vi "SacarNivelRefTablaRef.vi"(8 "error in (no error)":errorcluster, 11 "Prueba21 in":refnum<class "Prueba21.lvclass">) -> (0 "error out":errorcluster, 3 "Prueba21 out":refnum<class "Prueba21.lvclass">)   [LabVIEW 2019, in "Prueba21.lvclass"]
uses:
  Prueba21.lvclass
  Prueba21.lvclass/Prueba21.ctl
  Prueba/Prueba.lvclass
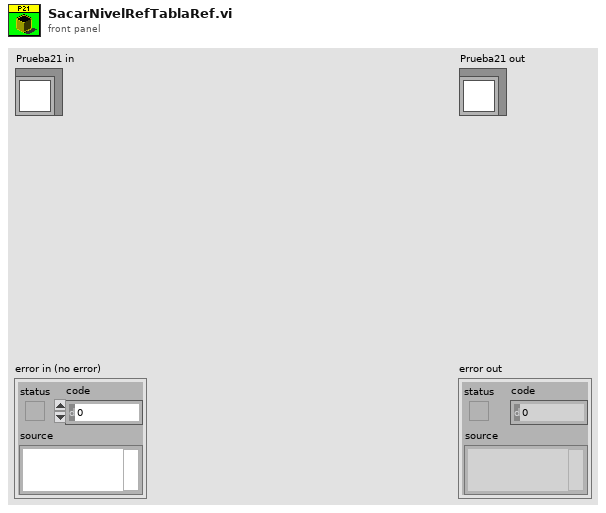
[diagram p1: front panel]
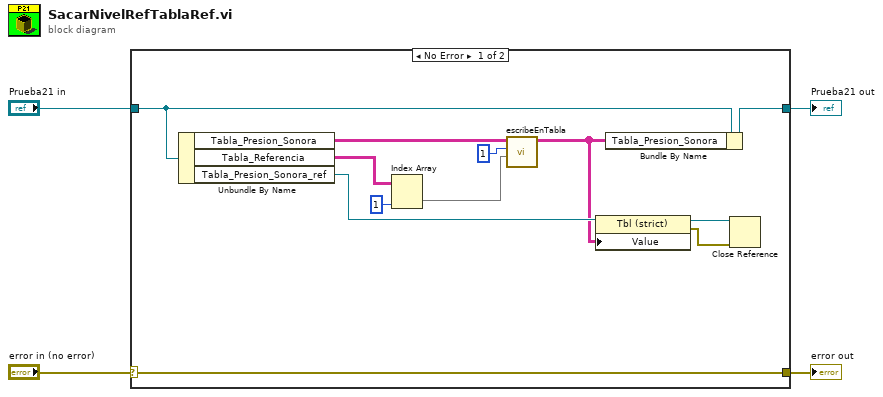
[diagram p0: block diagram]
diagram:
  n1 = case shown="No Error" "error in (no error)" {
    selector: "error in (no error)" -> [w16 w18]
    tunnel: [w16 w18] -> w3
    tunnel: [w9 w17] -> w1
    tunnel: "Prueba21 in" -> [w15 w17]
    frame No Error {
      n2 = Unbundle By Name(w15) -> ("Tabla_Presion_Sonora"=w11:string[][], "Tabla_Referencia"=w13:string[][], "Tabla_Presion_Sonora_ref"=w8:refnum<vi>)
      n3 = Index Array(array=w13, index (col)=1 ("disabled index (col)")) -> (element=w10:string[])  [unwired: 1 in]
      n4 = call "escribeEnTabla.vi"("parametros"=w10, "col"=1, "tabla in"=w11) -> ("tabla out"=w7:string[][])  [unwired: 8 in]
      n5 = property class="Tbl (strict)"(reference=w8, "Value"=w7) -> (reference out=w6:refnum<vi>, error out=w5:errorcluster)  [unwired: 1 in]
      n6 = Bundle By Name(cluster=w15, "Tabla_Presion_Sonora"=w7) -> (w9:refnum<class "Prueba21.lvclass">)
      n7 = Close Reference(reference=w6, error in (no error)=w5) -> ()  [unwired: 1 out]
    }
    frame Error {
    }
  }
  "error out" <- w3
  "Prueba21 out" <- w1
